vi "Start SubComponent.vi"(5 "Component ID":u8, 7 "FPGA Interface":refnum<class "FPGA Interface.lvclass">, 8 "error in (no error)":errorcluster, 11 "Remote Terminal in":refnum<class "Remote Terminal.lvclass">) -> (0 "error out":errorcluster, 3 "Remote Terminal out":refnum<class "Remote Terminal.lvclass">)   [LabVIEW 2020, in "BCI-1553 API.lvlib" / "Remote Terminal.lvclass"]
doc: "Ensures that the RemoteTerminal is enabled and then starts the operation of this Remote Terminal."
uses:
  Remote Terminal.lvclass
  Dependencies/FPGA Interface/FPGA Interface.lvclass
  Remote Terminal.lvclass/Remote Terminal.ctl
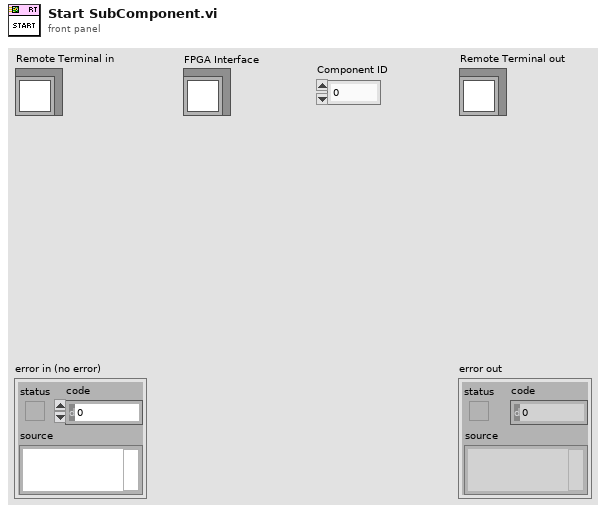
[diagram p1: front panel]
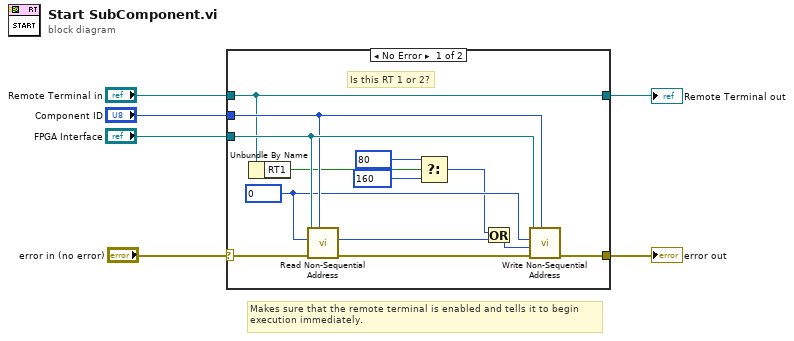
[diagram p0: block diagram]
diagram:
  # "Makes sure that the remote terminal is enabled and tells it to begin\nexecution immediately."
  n1 = case shown="No Error" "error in (no error)" {
    selector: "error in (no error)" -> [w17 w21]
    tunnel: [w15 w21] -> w1
    tunnel: "Remote Terminal in" -> [w9 w20]
    tunnel: "FPGA Interface" -> [w19 _]
    tunnel: "Component ID" -> [w18 _]
    tunnel: [w9 w20] -> w2
    frame No Error {
      w14 = u16 0 ("Address")
      # "Is this RT 1 or 2?"
      n2 = Unbundle By Name(w9) -> ("RT1"=w8:bool)
      n3 = call-dynamic "Read Non-Sequential Address.vi"("Target IC (1-8)"=w18, "error in (no error)"=w17, "Address"=w14, "FPGA Interface in"=w19) -> ("error out"=w16:errorcluster, "Data"=w13:u16)  [unwired: 6 in]
      n4 = Select(t=u16 80 ("Address"), s=w8, f=u16 160 ("Address")) -> (s? t:f=w10:u16)
      n5 = Or(x=w10, y=w13) -> (x .or. y?=w7:u16)
      n6 = call-dynamic "Write Non-Sequential Address.vi"("Target IC (1-8)"=w18, "error in (no error)"=w16, "Data"=w7, "Address"=w14, "FPGA Interface in"=w19) -> ("error out"=w15:errorcluster)  [unwired: 6 in]
    }
    frame Error {
    }
  }
  "error out" <- w1
  "Remote Terminal out" <- w2
